vi "Apply Package Name.vi"(8 "error in":errorcluster, 10 "Package Name":string, 11 "gRPC Message Metadata in":T1[](array[typedef])) -> (0 "error out":errorcluster, 3 "gRPC Message Metadata":T1[](array[typedef]))   [LabVIEW 2019, in "grpc-lvsupport.lvlib"]
uses:
  grpc-lvsupport.lvlib
  typeDefs/Message Element Type.ctl
  typeDefs/Message Element Metadata.ctl
  typeDefs/Message Metadata.ctl
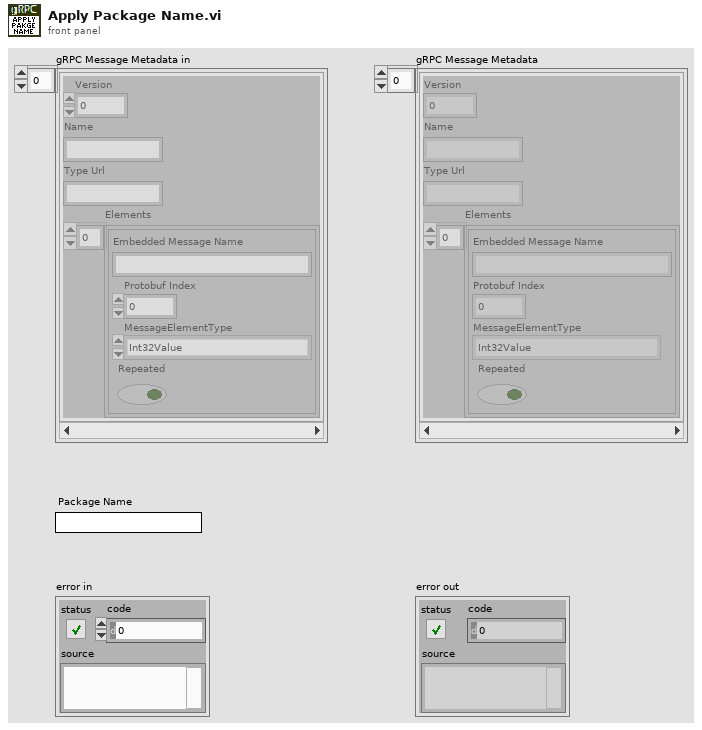
[diagram p1: front panel]
types:
  T1 = typedef "grpc-lvsupport.lvlib/Message Metadata.ctl" = cluster{"Version":i32, "Name":string, "Type Url":string, "Elements":T2[]}
  T2 = typedef "grpc-lvsupport.lvlib/Message Element Metadata.ctl" = cluster{"Embedded Message Name":string, "Protobuf Index":i32, "MessageElementType":T3, "Repeated":bool}
  T3 = typedef "grpc-lvsupport.lvlib/Message Element Type.ctl" = enum32{"Int32Value", "FloatValue", "DoubleValue", "BoolValue", "StringValue", "MessageValue", "Int64Value", "UInt32Value", "UInt64Value", "EnumValue", "Bytes", "Fixed64", "Fixed32", "SFixed64", "SFixed32", "SInt64", "SInt32"}
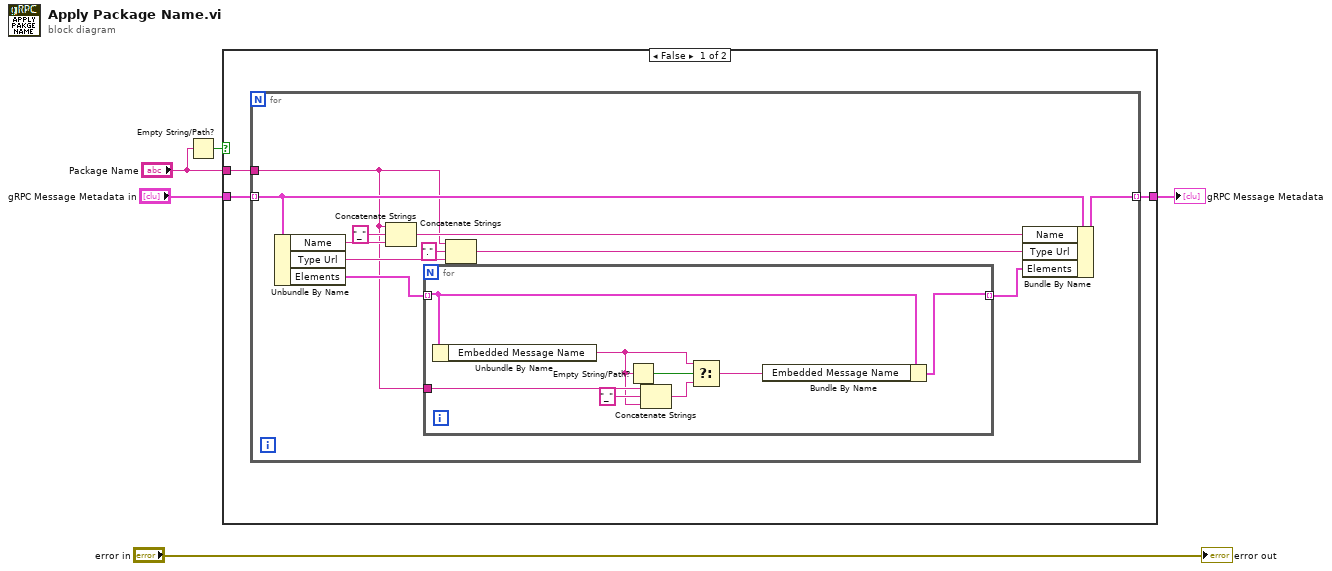
[diagram p0: block diagram]
diagram:
  n1 = Empty String/Path?(string/path="Package Name") -> (empty?=w1:bool)
  n2 = case shown="False" w1 {
    tunnel: "gRPC Message Metadata in" -> [w8 w28]
    tunnel: [w7 w28] -> w3
    tunnel: "Package Name" -> [w6 _]
    frame False {
      n3 = for {
        tunnel: w8 -> [w14] mode=indexing
        tunnel: w6 -> [w9]
        tunnel: [w11] -> w7 mode=indexing
        n4 = Unbundle By Name(w14) -> ("Name"=w18:string, "Type Url"=w15:string, "Elements"=w19:T2[])
        n5 = Concatenate Strings(w9, "_" ("string"), w18) -> (w13:string)
        n6 = for {
          tunnel: w19 -> [w24] mode=indexing
          tunnel: [w22] -> w10 mode=indexing
          tunnel: w9 -> [w21]
          n7 = Unbundle By Name(w24) -> ("Embedded Message Name"=w20:string)
          n8 = Empty String/Path?(string/path=w20) -> (empty?=w25:bool)
          n9 = Concatenate Strings(w21, "_" ("string"), w20) -> (w26:string)
          n10 = Select(t=w20, s=w25, f=w26) -> (s? t:f=w23:string)
          n11 = Bundle By Name(cluster=w24, "Embedded Message Name"=w23) -> (w22:T2)
        }
        n12 = Concatenate Strings(w9, "." ("string"), w15) -> (w12:string)
        n13 = Bundle By Name(cluster=w14, "Name"=w13, "Type Url"=w12, "Elements"=w10) -> (w11:T1)
      }
    }
    frame True {
    }
  }
  "gRPC Message Metadata" <- w3
  "error out" <- "error in"
